vi "SYST_PREF_ITEM_OFFS_RCV.vi"(0 "VISA IN":refnum<visa-resource-name>, 5 "error in":errorcluster, 7 "RxOffset":bool) -> (14 "VISA Out":refnum<visa-resource-name>, 19 "error out":errorcluster)   [LabVIEW 2018, in "PNA-X.lvlib"]
doc: "SYSTem:PREFerences:ITEM:OFFSet:RCV <bool> \n1876\n\n(Read-Write) Set and return whether to offset the test port receivers by the amount of receiver \nattenuation. Learn more. \nTo send this command using the PNA front panel, open the GPIB Command Processor Console, then \ntype either of the following examples at the command prompt. Then type the Query Syntax and press \nenter to be sure the PNA took the command. \nThis setting remains until changed again using this command, or until the hard drive is changed or \nreformatted. \nParameters \n<bool> Choose from: \nTrue (1) Offset the test port receivers \nFalse (0) Do NOT offset the test port receivers \nExamples SYST:PREF:ITEM:OFFS:RCV 1 \nsystem:preferences:item:offset:rcv false \nQuery Syntax SYSTem:PREFerences:ITEM:OFFSet:RCV? \nReturn Type Boolean \nDefault PNA-L and E836xB: False (does NOT offset the display). \nPNA-X: True (offsets the display)."
uses:
  PNA-X.lvlib
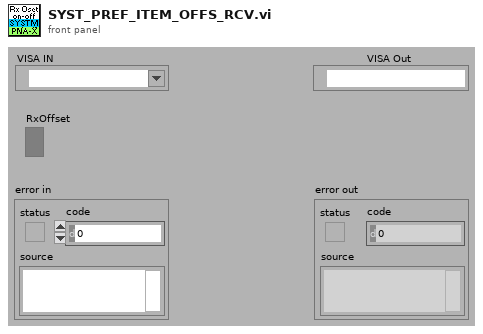
[diagram p1: front panel]
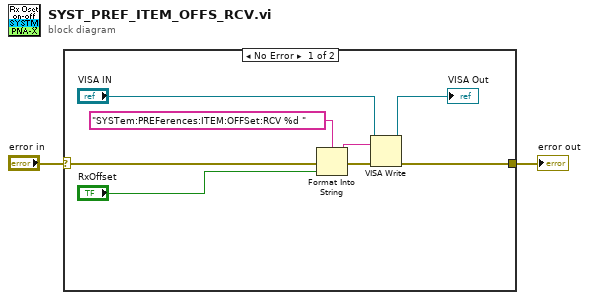
[diagram p0: block diagram]
diagram:
  n1 = case shown="No Error" "error in" {
    selector: "error in" -> [w10 w11]
    tunnel: [w5 w11] -> w1
    frame No Error {
      n2 = Format Into String(format string="SYSTem:PREFerences:ITEM:OFFSet:RCV %d " ("Cmdline"), error in=w10, "RxOffset") -> (resulting string=w8:string, error out=w9:errorcluster)  [unwired: 1 in]
      n3 = VISA Write(VISA resource name="VISA IN", write buffer=w8, error in (no error)=w9) -> (VISA resource name out=→"VISA Out":refnum<visa-resource-name>, error out=w5:errorcluster)  [unwired: 1 out]
    }
    frame Error {
    }
  }
  "error out" <- w1
